vi "Launch.vi"(8 "error in (no error)":errorcluster, 11 "Data Cluster In":T1={"Status"="", "SQLite"=refnum, "StationConfig"={"station_id"="", "schema_version"="", "sqlite_path"="", "syncagent_db_path"="", "postgres_conn"="", "sync_interval_sec"=0, "inbound_offset_sec"=0, "batch_size"=0, "table_overrides"=[]}, "OB Module ID"=-1, "IB Module ID"=-1, "is online"=FALSE, "CM alive?"=FALSE, "OB alive?"=FALSE, "IB alive?"=FALSE, "IB first cycle seen?"=FALSE, "OB first cycle seen?"=FALSE, "shutting down?"=FALSE, "exit code"=0, "status"=FALSE, "code"=0, "source"="", "ShutdownReason"=enum."None", "OB last cycle at"=timestamp(0 s since 1904-01-01), "IB last cycle at"=timestamp(0 s since 1904-01-01), "Baseline Config"={"Baseline Mode"=enum."None", "From Date"="", "Chunk Size"=1000, "Verify Checksums"=TRUE}}) -> (0 "error out":errorcluster, 3 "Data Cluster Out":T1={"Status"="", "SQLite"=refnum, "StationConfig"={"station_id"="", "schema_version"="", "sqlite_path"="", "syncagent_db_path"="", "postgres_conn"="", "sync_interval_sec"=0, "inbound_offset_sec"=0, "batch_size"=0, "table_overrides"=[]}, "OB Module ID"=-1, "IB Module ID"=-1, "is online"=FALSE, "CM alive?"=FALSE, "OB alive?"=FALSE, "IB alive?"=FALSE, "IB first cycle seen?"=FALSE, "OB first cycle seen?"=FALSE, "shutting down?"=FALSE, "exit code"=0, "status"=FALSE, "code"=0, "source"="", "ShutdownReason"=enum."None", "OB last cycle at"=timestamp(0 s since 1904-01-01), "IB last cycle at"=timestamp(0 s since 1904-01-01), "Baseline Config"={"Baseline Mode"=enum."None", "From Date"="", "Chunk Size"=1000, "Verify Checksums"=TRUE}})   [LabVIEW 2025, in "Dashboard.lvlib"]
uses:
  Dashboard.lvlib
  OpCore/SQLite/SQLite.lvclass
  OpCore/Libraries/Connection Monitor/Connection Monitor.lvlib
  OpCore/Libraries/Inbound Sync/Inbound Sync.lvlib
  OpCore/Libraries/Outbound Sync/Outbound Sync.lvlib
  OpCore/OpCore Types/SyncDirection.ctl
  OpCore/OpCore Types/OpCore Types.lvlib
  OpCore/OpCore Types/TableOverride.ctl
  OpCore/OpCore Types/StationConfig.ctl
  OpCore/OpCore Types/ShutdownReason.ctl
  OpCore/OpCore Types/BaselineMode.ctl
  OpCore/OpCore Types/Baseline Config.ctl
  Module Data--cluster.ctl
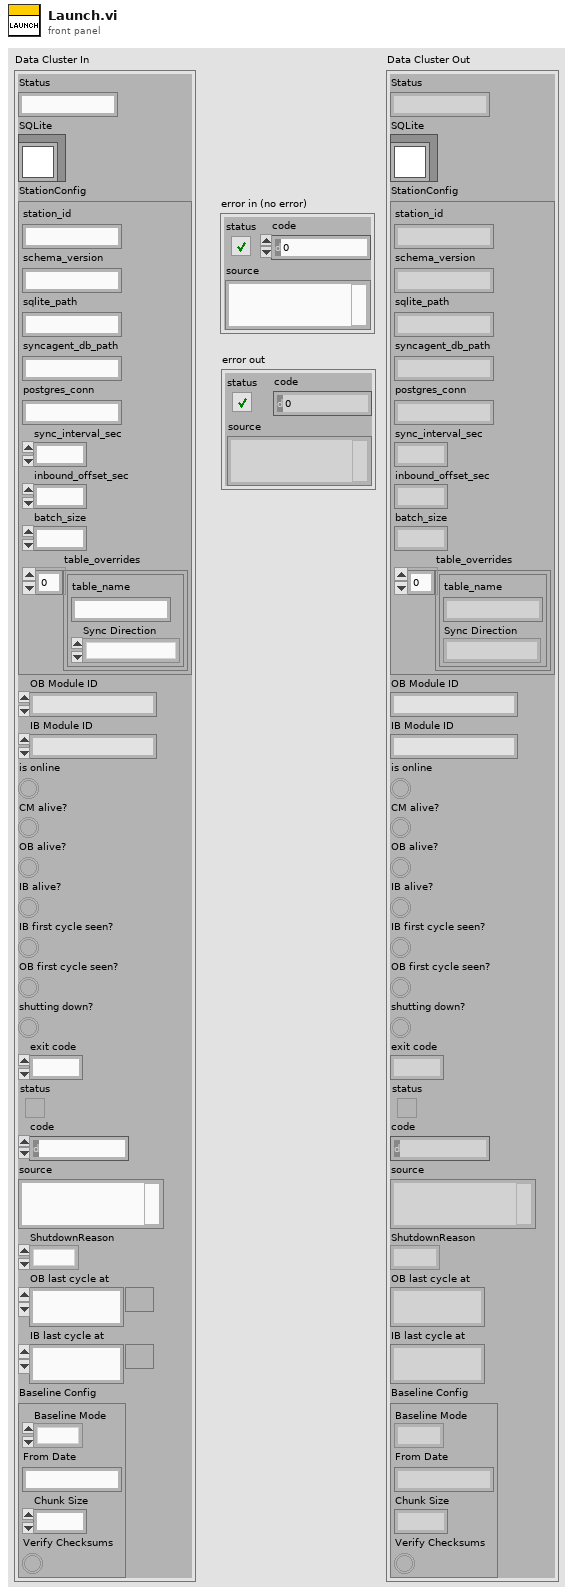
[diagram p1: front panel]
types:
  T1 = typedef "Dashboard.lvlib/Module Data--cluster.ctl" = cluster{"Status":string, "SQLite":refnum<class "SQLite.lvclass">, "StationConfig":T2, "OB Module ID":i32, "IB Module ID":i32, "is online":bool, "CM alive?":bool, "OB alive?":bool, "IB alive?":bool, "IB first cycle seen?":bool, "OB first cycle seen?":bool, "shutting down?":bool, "exit code":i32, "status":bool, "code":i32, "source":string, "ShutdownReason":T5, "OB last cycle at":timestamp, "IB last cycle at":timestamp, "Baseline Config":T6}
  T2 = typedef "OpCore Types.lvlib/StationConfig.ctl" = cluster{"station_id":string, "schema_version":string, "sqlite_path":string, "syncagent_db_path":string, "postgres_conn":string, "sync_interval_sec":i32, "inbound_offset_sec":i32, "batch_size":i32, "table_overrides":T3[]}
  T3 = typedef "OpCore Types.lvlib/TableOverride.ctl" = cluster{"table_name":string, "Sync Direction":T4}
  T4 = typedef "OpCore Types.lvlib/SyncDirection.ctl" = enum16{"Both", "Outbound_Only", "Inbound_Only", "Exclude"}
  T5 = typedef "OpCore Types.lvlib/ShutdownReason.ctl" = enum16{"None", "Operator", "Service", "ModuleDied", "Fatal"}
  T6 = typedef "OpCore Types.lvlib/Baseline Config.ctl" = cluster{"Baseline Mode":T7, "From Date":string, "Chunk Size":i32, "Verify Checksums":bool}
  T7 = typedef "OpCore Types.lvlib/BaselineMode.ctl" = enum16{"None", "Full", "From Date"}
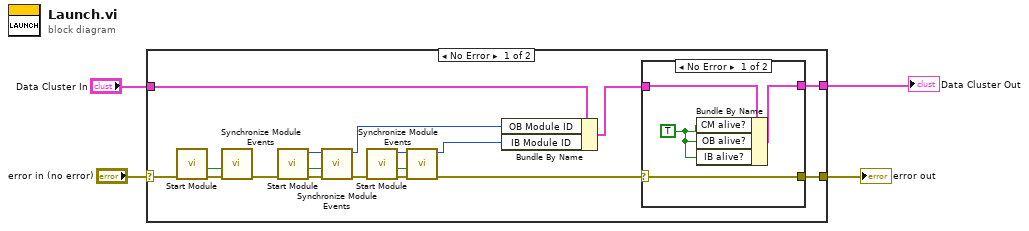
[diagram p0: block diagram]
diagram:
  n1 = case shown="No Error" "error in (no error)" {
    selector: "error in (no error)" -> [w19 w30]
    tunnel: [w11 w30] -> w3
    tunnel: "Data Cluster In" -> [w9 w29]
    tunnel: [w10 w29] -> w1
    frame No Error {
      n2 = call "Start Module.vi"("error in"=w19) -> ("error out"=w22:errorcluster, "Wait for Event Sync?"=w18:bool)  [unwired: 6 in, 3 out]
      n3 = call "Synchronize Module Events.vi"("error in"=w22, "Wait for Event Sync?"=w18) -> ("error out"=w7:errorcluster)  [unwired: 9 in]
      n4 = call "Start Module.vi"("error in"=w7) -> ("error out"=w21:errorcluster, "Wait for Event Sync?"=w17:bool, "Module ID"=w15:i32)  [unwired: 6 in, 2 out]
      n5 = call "Synchronize Module Events.vi"("error in"=w21, "Wait for Event Sync?"=w17, "Module ID in"=w15) -> ("error out"=w6:errorcluster, "Module ID out"=w13:i32)  [unwired: 7 in]
      n6 = call "Start Module.vi"("error in"=w6) -> ("error out"=w20:errorcluster, "Wait for Event Sync?"=w16:bool, "Module ID"=w14:i32)  [unwired: 6 in, 2 out]
      n7 = call "Synchronize Module Events.vi"("error in"=w20, "Wait for Event Sync?"=w16, "Module ID in"=w14) -> ("error out"=w5:errorcluster, "Module ID out"=w12:i32)  [unwired: 7 in]
      n8 = Bundle By Name(cluster=w9, "OB Module ID"=w13, "IB Module ID"=w12) -> (w8:T1)
      n9 = case shown="No Error" w5 {
        selector: w5 -> [w26 w28]
        tunnel: [w26 w28] -> w11
        tunnel: w8 -> [w24 w27]
        tunnel: [w23 w27] -> w10
        frame No Error {
          w25 = TRUE ("CM alive?")
          n10 = Bundle By Name(cluster=w24, "CM alive?"=w25, "OB alive?"=w25, "IB alive?"=w25) -> (w23:T1)
        }
        frame Error {
        }
      }
    }
    frame Error {
    }
  }
  "error out" <- w3
  "Data Cluster Out" <- w1
